vi "detectAllVarables.vi"(3 "error in (no error)":errorcluster, 5 "VISA resource name":refnum<visa-resource-name>="COM1" caption="端口号") -> (0 "error out":errorcluster, 1 "Data":T1[](array[typedef]), 2 "VISA resource name 2":refnum<visa-resource-name>="COM1" caption="端口号")   [LabVIEW 2010]
uses:
  OutputDataFormat.ctl
  GlobalCostants.vi
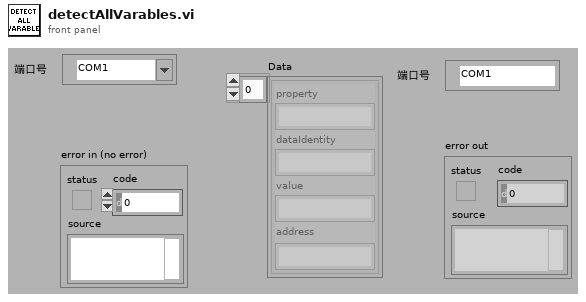
[diagram p1: front panel]
types:
  T1 = typedef "OutputDataFormat.ctl" = cluster{"property":string, "dataIdentity":string, "value":string, "address":string}
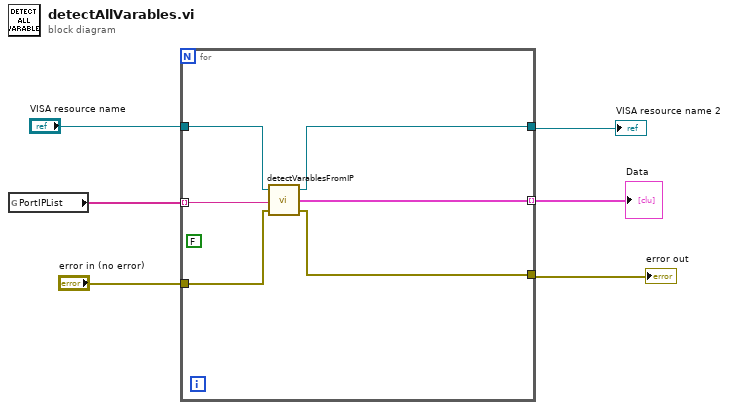
[diagram p0: block diagram]
diagram:
  n1 = global read "GlobalCostants.vi" "PortIPList"() -> (w2:string[])
  n2 = for {
    tunnel: [w12] -> w6
    tunnel: [w11] -> w1 mode=indexing
    tunnel: [w10] -> w5
    tunnel: "error in (no error)" -> [w9]
    tunnel: "VISA resource name" -> [w8]
    tunnel: w2 -> [w7] mode=indexing
    (unwired) FALSE
    n3 = call "detectVarablesFromIP.vi"("error in (no error)"=w9, "PortIP"=w7, "VISA resource name"=w8) -> ("error out"=w10:errorcluster, "Data"=w11:T1, "VISA resource name 2"=w12:refnum<visa-resource-name>)
  }
  "VISA resource name 2" <- w6
  "error out" <- w5
  "Data" <- w1
